vi "TestServerStreaming.vi"() -> ()   [LabVIEW 2019]
uses:
  Servers/TestDataMarshal/TestDataMarshal Class/RPC Messages/queryserver_ServerEvent/queryserver_ServerEvent_Data.ctl
  b86462cc-b845-42fe-a1c6-22aba0980919.vi
  cc31af3b-fcb0-4882-9b4f-6fb24e2d67b3.vi
  labview source/gRPC lv Support/Server API/Server/Get Server DLL Path.vi
  labview source/gRPC lv Support/gprc-lvsupport.lvlib
  Servers/TestDataMarshal/TestDataMarshal Class/TestDataMarshal.lvclass
panel:
  out "Response Data":T1
  out "Numeric":i32
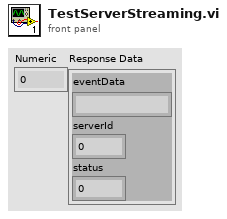
[diagram p1: front panel]
types:
  T1 = typedef "TestDataMarshal.lvlib/TestDataMarshal.lvclass/queryserver_ServerEvent_Data.ctl" = cluster{"eventData":string, "serverId":i32, "status":i32}
  T2 = typedef "gprc-lvsupport.lvlib/grpcId.ctl" = u64
  T3 = typedef "TestDataMarshal.lvlib/gprc-lvsupport.lvlib/grpcId.ctl" = u64
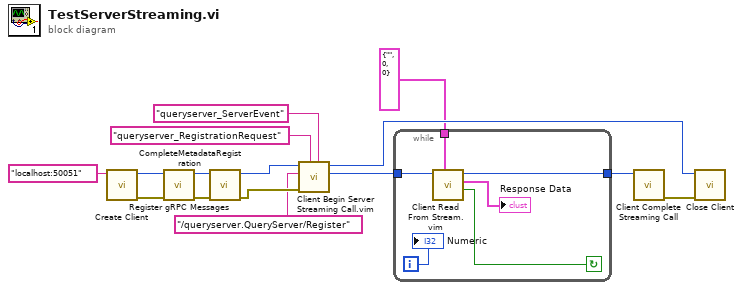
[diagram p0: block diagram]
diagram:
  n1 = call "Create Client.vi"("address"="localhost:50051") -> ("error out"=w7:errorcluster, "Client Ref Out"=w15:T2)  [unwired: 9 in]
  n2 = call "Register gRPC Messages.vi"("error in (no error)"=w7, "gRPC ID"=w15) -> ("error out"=w6:errorcluster, "gRPC ID Out"=w14:T3)  [unwired: 8 in]
  n3 = call "CompleteMetadataRegistration.vi"("error in (no error)"=w6, "gRPC ID"=w14) -> ("error out"=w5:errorcluster, "gRPC ID Out"=w12:T2)  [unwired: 8 in]
  n4 = call "Client Begin Server Streaming Call.vim"("Response Message Name"="queryserver_ServerEvent", "Request Message Name"="queryserver_RegistrationRequest", "error in (no error)"=w5, "Method Name"="/queryserver.QueryServer/Register", "Client Ref"=w12) -> ("Call Id Out"=w10:u64, "Client Ref Out"=w9:u64)  [unwired: 4 in, 1 out]
  n5 = while {
    tunnel: [w21] -> w11
    tunnel: w10 -> [w19]
    tunnel: T1 {"eventData"="", "serverId"=0, "status"=0} ("queryserver_ServerEvent_Data") -> [w18]
    i -> [w20]
    stop <- w16 continue-if-true
    n6 = call "Client Read From Stream.vim"("Response Type"=w18, "Call Id in"=w19) -> ("Success"=w16:bool, "Response Data"=→"Response Data":T1, "Call Id Out"=w21:u64)  [unwired: 6 in, 1 out]
    "Numeric" <- w20
  }
  n7 = call "Client Complete Streaming Call.vi"("Call Id"=w11) -> ("error out"=w8:errorcluster)  [unwired: 9 in, 1 out]
  n8 = call "Close Client.vi"("error in (no error)"=w8, "Client Ref"=w9) -> ()  [unwired: 9 in, 1 out]
